vi "Write Data File.lvclass.vi"(8 "error in (no error)":errorcluster, 10 "Abstruct Data Type.lvclass":refnum<class "Abstruct Data Type.lvclass">, 11 "Data Loader in":refnum<class "Data Loader.lvclass">) -> (0 "error out":errorcluster, 3 "Data Loader out":refnum<class "Data Loader.lvclass">)   [LabVIEW 2020, in "Data Loader.lvlib" / "Data Loader.lvclass"]
uses:
  Data Loader.lvclass
  Data Types/Abstrut Data/Abstruct Data Type.lvclass
  Data Loader.lvclass/Data Loader.ctl
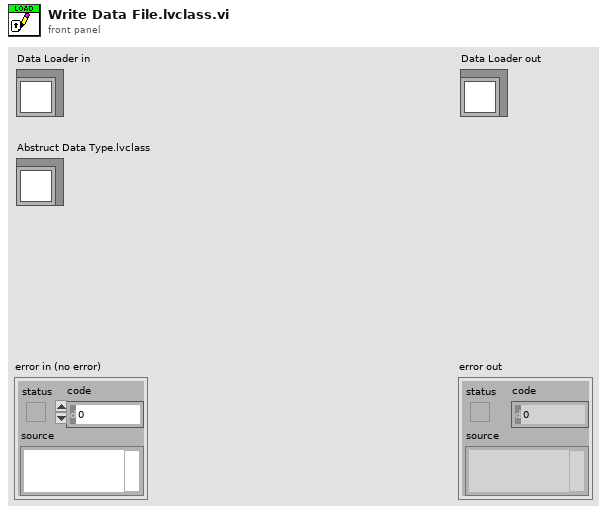
[diagram p1: front panel]
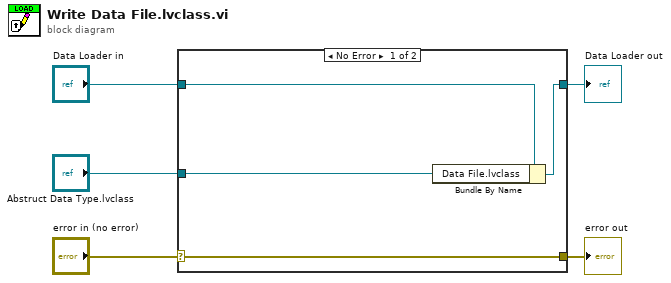
[diagram p0: block diagram]
diagram:
  n1 = case shown="No Error" "error in (no error)" {
    selector: "error in (no error)" -> [w9 w10]
    tunnel: [w9 w10] -> w4
    tunnel: [w7 w11] -> w2
    tunnel: "Data Loader in" -> [w8 w11]
    tunnel: "Abstruct Data Type.lvclass" -> [w6 _]
    frame No Error {
      n2 = Bundle By Name(cluster=w8, "Data File.lvclass"=w6) -> (w7:refnum<class "Data Loader.lvclass">)
    }
    frame Error {
    }
  }
  "error out" <- w4
  "Data Loader out" <- w2
